vi "NT Read Generic Value.vi"(6 "type variant":variant, 8 "error in":errorcluster, 9 "Add Name":bool, 11 "name":string="Boolean") -> (0 "error out":errorcluster, 3 "variant value":variant)   [LabVIEW 2025]
doc: "Return the tagged cluster data for the named entry."
uses:
  <vilib>/Rock Robotics/Network Tables/NT SubscribeOptions.ctl
  <vilib>/Rock Robotics/Network Tables/NT Datatype.ctl
  ntcoreffi.dll
panel:
  out "timestamp":u64
  in  "description":string="boolean"
  in  "options":T1={"Send All"=FALSE, "Keep Duplicates"=FALSE, "rate (hz)"=10}
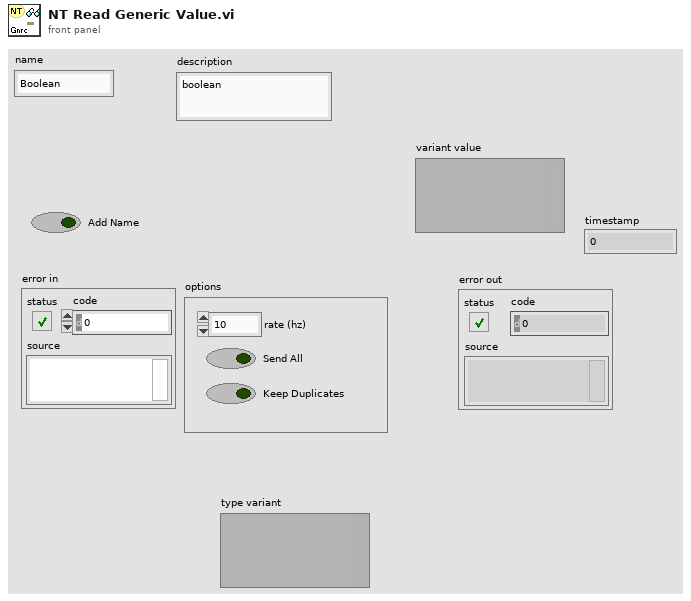
[diagram p1: front panel]
types:
  T1 = typedef "NT SubscribeOptions.ctl" = cluster{"Send All":bool, "Keep Duplicates":bool, "rate (hz)":u64}
  T2 = typedef "NT Datatype.ctl" = u32
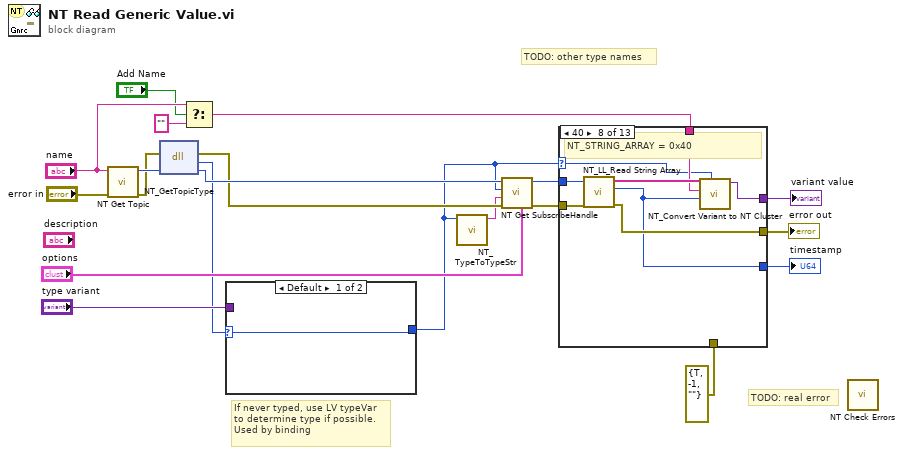
[diagram p0: block diagram]
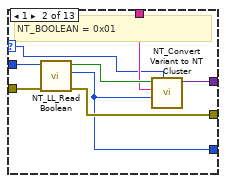
[diagram p3: hidden frame]
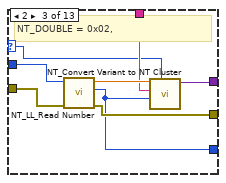
[diagram p4: hidden frame]
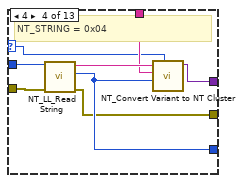
[diagram p5: hidden frame]
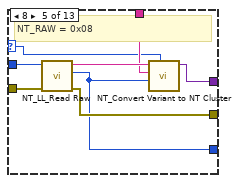
[diagram p6: hidden frame]
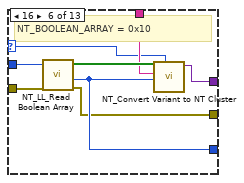
[diagram p7: hidden frame]
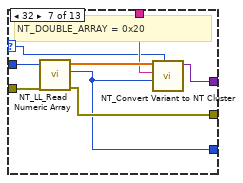
[diagram p8: hidden frame]
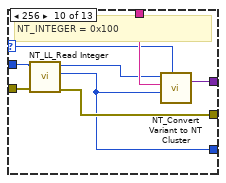
[diagram p10: hidden frame]
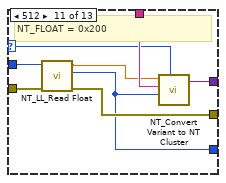
[diagram p11: hidden frame]
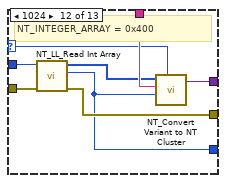
[diagram p12: hidden frame]
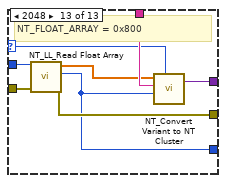
[diagram p13: hidden frame]
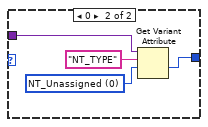
[diagram p14: hidden frame]
diagram:
  # "If never typed, use LV typeVar\nto determine type if possible.\nUsed by binding"
  # "TODO: other type names"
  # "TODO: real error"
  n1 = call <vilib>:"NT Get Topic.vi"("error in (no error)"="error in", "name"="name") -> ("error out"=w16:errorcluster, "topicHandle"=w19:u32)  [unwired: 8 in]
  n2 = dll-call lib="ntcoreffi.*" fn="NT_GetTopicType"(error in=w16, "topic"=w19) -> (error out=w15:errorcluster, "type"=w2:u32, "topic"=w18:u32)  [unwired: 2 in, 1 out]
  n3 = Select(t="name", s="Add Name", f="") -> (s? t:f=w6:string)
  n4 = case shown="Default" w2 {
    selector: w2 -> [w21 _]
    tunnel: "type variant" -> [_ w23]
    tunnel: [w21 w22] -> w1
    frame Default {
    }
    frame 0 {
      w25 = T2 0 items=["NT_Unassigned"=0, "NT_Boolean"=1, "NT_Double"=2, "NT_String"=4, "NT_Raw"=8, "NT_BooleanArray"=16, "NT_DoubleArray"=32, "NT_StringArray"=64, "NT_RPC"=128, "NT_Integer"=256, "NT_Float"=512, "NT_IntegerArray"=1024, "NT_FloatArray"=2048] ("NT_Type")
      n5 = Get Variant Attribute(Variant=w23, name="NT_TYPE", default value (empty Variant)=w25) -> (value=w22:T2)  [unwired: 1 in, 3 out]
    }
  }
  n6 = call <vilib>:"NT_TypeToTypeStr.vi"("type"=w1) -> ("typeStr"=w4:string)  [unwired: 10 in]
  n7 = call <vilib>:"NT Get SubscribeHandle.vi"("options"="options", "error in (no error)"=w15, "description"=w4, "NT_Type"=w1, "topicHandle"=w18) -> ("error out"=w14:errorcluster, "subscribeHandle"=w13:u32)  [unwired: 5 in]
  n8 = case shown="40" w1 {
    selector: w1 -> [_ w27 w35 w43 w51 w59 w67 w75 _ w85 w93 w101 w109]
    tunnel: w14 -> [_ w30 w41 w49 w57 w65 w73 w81 _ w90 w96 w104 w112]
    tunnel: errorcluster {"status"=TRUE, "code"=-1, "source"=""} ("error out") -> [w26 _ _ _ _ _ _ _ w83 _ _ _ _]
    tunnel: w13 -> [_ w34 w42 w50 w58 w66 w74 w82 _ w91 w97 w105 w113]
    tunnel: [_ w32 w38 w45 w55 w61 w70 w78 _ w89 w99 w107 w115] -> w12
    tunnel: [w26 w31 w39 w46 w54 w62 w71 w79 w83 w86 w94 w102 w110] -> w11
    tunnel: [_ w29 w37 w47 w53 w63 w69 w77 _ w84 w92 w100 w108] -> w9
    tunnel: w6 -> [_ w28 w36 w44 w52 w60 w68 w76 _ w88 w98 w106 w114]
    frame 0, Default {
      # "NT_UNASSIGNED=0"
    }
    frame 1 {
      # "NT_BOOLEAN = 0x01"
      n9 = call <vilib>:"NT_LL_Read Boolean.vi"("error in (no error)"=w30, "subscribeHandle"=w34) -> ("error out"=w31:errorcluster, "time"=w29:i64, "Boolean"=w33:bool)  [unwired: 7 in]
      n10 = call <vilib>:"NT_Convert Variant to NT Cluster.vi"("NT_Type"=w27, "timestamp"=w29, "Name"=w28, "NewVal"=w33) -> ("Value out"=w32:variant)  [unwired: 6 in, 1 out]
    }
    frame 2 {
      # "NT_DOUBLE = 0x02,"
      n11 = call <vilib>:"NT_LL_Read Number.vi"("error in (no error)"=w41, "subscribeHandle"=w42) -> ("error out"=w39:errorcluster, "time"=w37:i64, "value"=w40:dbl)  [unwired: 7 in]
      n12 = call <vilib>:"NT_Convert Variant to NT Cluster.vi"("NT_Type"=w35, "timestamp"=w37, "Name"=w36, "NewVal"=w40) -> ("Value out"=w38:variant)  [unwired: 6 in, 1 out]
    }
    frame 4 {
      # "NT_STRING = 0x04"
      n13 = call <vilib>:"NT_LL_Read String.vi"("error in (no error)"=w49, "subscribeHandle"=w50) -> ("error out"=w46:errorcluster, "time"=w47:i64, "value"=w48:string)  [unwired: 7 in]
      n14 = call <vilib>:"NT_Convert Variant to NT Cluster.vi"("NT_Type"=w43, "timestamp"=w47, "Name"=w44, "NewVal"=w48) -> ("Value out"=w45:variant)  [unwired: 6 in, 1 out]
    }
    frame 8 {
      # "NT_RAW = 0x08"
      n15 = call <vilib>:"NT_LL_Read Raw.vi"("error in (no error)"=w57, "subscribeHandle"=w58) -> ("error out"=w54:errorcluster, "time"=w53:i64, "string"=w56:string)  [unwired: 7 in]
      n16 = call <vilib>:"NT_Convert Variant to NT Cluster.vi"("NT_Type"=w51, "timestamp"=w53, "Name"=w52, "NewVal"=w56) -> ("Value out"=w55:variant)  [unwired: 6 in, 1 out]
    }
    frame 16 {
      # "NT_BOOLEAN_ARRAY = 0x10"
      n17 = call <vilib>:"NT_LL_Read Boolean Array.vi"("error in (no error)"=w65, "subscribeHandle"=w66) -> ("error out"=w62:errorcluster, "server time"=w63:i64, "value"=w64:bool[])  [unwired: 6 in, 1 out]
      n18 = call <vilib>:"NT_Convert Variant to NT Cluster.vi"("NT_Type"=w59, "timestamp"=w63, "Name"=w60, "NewVal"=w64) -> ("Value out"=w61:variant)  [unwired: 6 in, 1 out]
    }
    frame 32 {
      # "NT_DOUBLE_ARRAY = 0x20"
      n19 = call <vilib>:"NT_LL_Read Numeric Array.vi"("error in (no error)"=w73, "subscribeHandle"=w74) -> ("error out"=w71:errorcluster, "time"=w69:i64, "value"=w72:dbl[])  [unwired: 7 in]
      n20 = call <vilib>:"NT_Convert Variant to NT Cluster.vi"("NT_Type"=w67, "timestamp"=w69, "Name"=w68, "NewVal"=w72) -> ("Value out"=w70:variant)  [unwired: 6 in, 1 out]
    }
    frame 64 {
      # "NT_STRING_ARRAY = 0x40"
      n21 = call <vilib>:"NT_LL_Read String Array.vi"("error in"=w81, "subscribeHandle"=w82) -> ("error out"=w79:errorcluster, "time"=w77:i64, "value"=w80:string[])  [unwired: 7 in]
      n22 = call <vilib>:"NT_Convert Variant to NT Cluster.vi"("NT_Type"=w75, "timestamp"=w77, "Name"=w76, "NewVal"=w80) -> ("Value out"=w78:variant)  [unwired: 6 in, 1 out]
    }
    frame 128 {
      # "NT_RPC = 0x80"
    }
    frame 256 {
      # "NT_INTEGER = 0x100"
      n23 = call <vilib>:"NT_LL_Read Integer.vi"("error in (no error)"=w90, "subscribeHandle"=w91) -> ("error out"=w86:errorcluster, "time"=w84:i64, "value"=w87:i64)  [unwired: 7 in]
      n24 = call <vilib>:"NT_Convert Variant to NT Cluster.vi"("NT_Type"=w85, "timestamp"=w84, "Name"=w88, "NewVal"=w87) -> ("Value out"=w89:variant)  [unwired: 6 in, 1 out]
    }
    frame 512 {
      # "NT_FLOAT = 0x200"
      n25 = call <vilib>:"NT_LL_Read Float.vi"("error in (no error)"=w96, "subscribeHandle"=w97) -> ("error out"=w94:errorcluster, "time"=w92:i64, "value"=w95:sgl)  [unwired: 7 in]
      n26 = call <vilib>:"NT_Convert Variant to NT Cluster.vi"("NT_Type"=w93, "timestamp"=w92, "Name"=w98, "NewVal"=w95) -> ("Value out"=w99:variant)  [unwired: 6 in, 1 out]
    }
    frame 1024 {
      # "NT_INTEGER_ARRAY = 0x400"
      n27 = call <vilib>:"NT_LL_Read Int Array.vi"("error in (no error)"=w104, "subscribeHandle"=w105) -> ("error out"=w102:errorcluster, "time"=w100:i64, "value"=w103:i64[])  [unwired: 7 in]
      n28 = call <vilib>:"NT_Convert Variant to NT Cluster.vi"("NT_Type"=w101, "timestamp"=w100, "Name"=w106, "NewVal"=w103) -> ("Value out"=w107:variant)  [unwired: 6 in, 1 out]
    }
    frame 2048 {
      # "NT_FLOAT_ARRAY = 0x800"
      n29 = call <vilib>:"NT_LL_Read Float Array.vi"("error in (no error)"=w112, "subscribeHandle"=w113) -> ("error out"=w110:errorcluster, "time"=w108:i64, "value"=w111:sgl[])  [unwired: 7 in]
      n30 = call <vilib>:"NT_Convert Variant to NT Cluster.vi"("NT_Type"=w109, "timestamp"=w108, "Name"=w114, "NewVal"=w111) -> ("Value out"=w115:variant)  [unwired: 6 in, 1 out]
    }
  }
  "error out" <- w11
  "variant value" <- w12
  "timestamp" <- w9
  n31 = call <vilib>:"NT Check Errors.vi"() -> ()  [unwired: 11 in, 1 out]
